vi "Shooter_Equation.vi"(10 "Right Trigger":dbl, 11 "Ty":dbl) -> (3 "% voltage":dbl)   [LabVIEW 2020]
uses:
  <vilib>/Rock Robotics/WPI/ThirdParty/Phoenix-LabVIEW/Motor Controller/Controls/CTRE_Phoenix_MotorControl_ControlMode.ctl
  <vilib>/Rock Robotics/Network Tables/NT Read Number.vi
  <vilib>/Rock Robotics/Network Tables/NT Write Number.vi
panel:
  out "voltage (V)":dbl
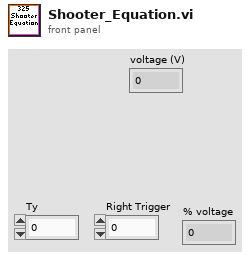
[diagram p1: front panel]
types:
  T1 = typedef "CTRE_Phoenix_MotorControl_ControlMode.ctl" = u16
  T2 = typedef "WPI_MotorControlDeviceRef.ctl" = cluster{"DeviceStatus":errorcluster, "Type":T3, "PWM":cluster{"PWM Channel":T4, "DeadBand":T5}, "CAN":cluster{"Device Number":u8, "SetOutput VI Ref":variant, "GetOutput VI Ref":variant, "Enable VI Ref":variant, "Disable VI Ref":variant, "Data":variant}, "Invert":bool, "DIO PWM":cluster{"PWM \"Enable\" Channel":T4, "DIOChannel":T6, "PWM Rate":dbl}}
  T3 = typedef "WPI_MotorControlType.ctl" = enum16{"PWM", "CAN", "DIO PWM"}
  T4 = typedef "FPGA_DIOPWMChannel.ctl" = enum8{"PWM 0", "PWM 1", "PWM 2", "PWM 3", "PWM 4", "PWM 5", "PWM 6", "PWM 7", "PWM 8", "PWM 9", "PWM MXP 0", "PWM MXP 1", "PWM MXP 2", "PWM MXP 3", "PWM MXP 4", "PWM MXP 5", "PWM MXP 6", "PWM MXP 7", "PWM MXP 8", "PWM MXP 9", "Invalid"}
  T5 = typedef "WPI_PWMDeadband.ctl" = cluster{"Name":string, "maxPositivePwm":i32, "minPositivePwm":i32, "centerPwm":i32, "maxNegativePwm":i32, "minNegativePwm":i32, "angularRange":u16}
  T6 = typedef "FPGA_DIOChannel.ctl" = enum8{"DIO 0", "DIO 1", "DIO 2", "DIO 3", "DIO 4", "DIO 5", "DIO 6", "DIO 7", "DIO 8", "DIO 9", "DIO MXP 0", "DIO MXP 1", "DIO MXP 2", "DIO MXP 3", "DIO MXP 4", "DIO MXP 5", "DIO MXP 6", "DIO MXP 7", "DIO MXP 8", "DIO MXP 9", "DIO MXP 10", "DIO MXP 11", "DIO MXP 12", "DIO MXP 13", "DIO MXP 14", "DIO MXP 15", "SPI Port CS1", "SPI Port CS2", "SPI Port CS3", "SPI Port MISO", "SPI Port MOSI", "Invalid"}
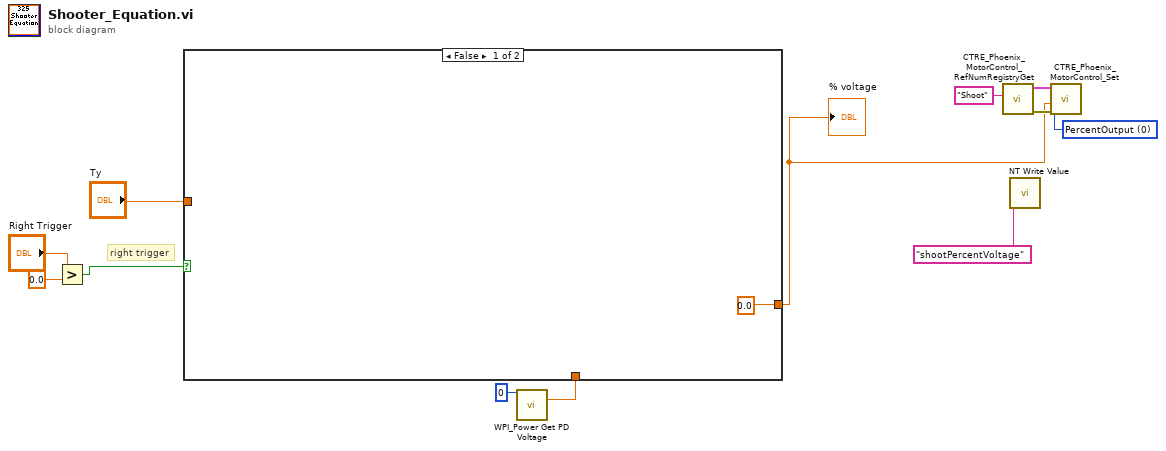
[diagram p0: block diagram]
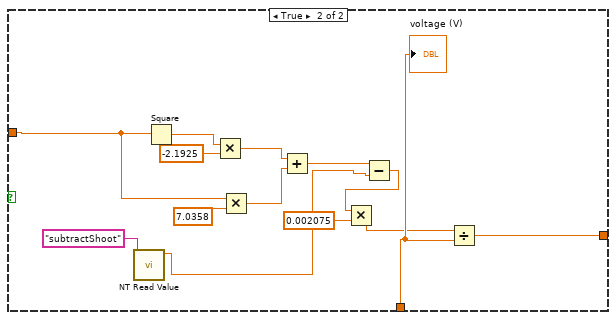
[diagram p2: hidden frame]
diagram:
  w6 = T1 0 items=["PercentOutput"=0, "Position"=1, "Velocity"=2, "Current"=3, "Follower"=5, "MotionProfile"=6, "MotionMagic"=7, "MotionProfileArc"=10, "Disabled"=15] ("Control Mode")
  # "right trigger"
  n1 = Greater?(x="Right Trigger", y=0.0) -> (0:w4:bool)
  n2 = call <vilib>:"WPI_Power Get PD Voltage.vi"("Power Distribution Panel (def)"=u8 0) -> ("voltage (V)"=w11:dbl)  [unwired: 13 in, 1 out]
  n3 = case shown="False" w4 {
    tunnel: "Ty" -> [_ w24]
    tunnel: w11 -> [_ w18]
    tunnel: [0.0 ("Shoot %") w16] -> w1
    frame False {
    }
    frame True {
      n4 = call-poly <vilib>:"NT Read Value.vi"("Name"="subtractShoot") -> ("Numeric"=w15:dbl)  [unwired: 9 in, 1 out]
      n5 = Square(x=w24) -> (x^2=w27:dbl)
      n6 = Multiply(x=w27, y=-2.1925) -> (x*y=w25:dbl)
      n7 = Multiply(x=w24, y=7.0358) -> (x*y=w22:dbl)
      n8 = Add(x=w25, y=w22) -> (x+y=w21:dbl)
      n9 = Subtract(x=w21, y=w15) -> (x-y=w20:dbl)
      n10 = Multiply(x=w20, y=0.002075) -> (x*y=w17:dbl)
      n11 = Divide(x=w17, y=w18) -> (x/y=w16:dbl)
      "voltage (V)" <- w18
    }
  }
  "% voltage" <- w1
  n12 = call <vilib>:"CTRE_Phoenix_MotorControl_RefNumRegistryGet.vi"("refnum name"="Shoot") -> ("error out"=w9:errorcluster, "PhoenixMotorControlDevRef"=w8:T2)  [unwired: 9 in]
  n13 = call-poly <vilib>:"NT Write Value.vi"("Name"="shootPercentVoltage") -> ()  [unwired: 10 in, 1 out]
  n14 = call <vilib>:"CTRE_Phoenix_MotorControl_Set.vi"("error in (no error)"=w9, "Output"=w1, "Control Mode"=w6, "PhoenixMotorControlDevRef"=w8) -> ()  [unwired: 6 in, 2 out]
